vi "proba_3.vi"() -> ()   [LabVIEW 2015]
uses:
  <vilib>/MakerHub/LINX/Public/Peripherals/Digital/Digital Write N Chans.vi
  <vilib>/MakerHub/LINX/Public/Peripherals/Analog/Analog Read 1 Chan.vi
  <vilib>/MakerHub/LINX/Private/Local IO/LinxDigitalWrite.vi
  <vilib>/MakerHub/LINX/Public/Utilities/Check Channel.vi
  <vilib>/MakerHub/LINX/Public/Peripherals/Analog/Analog Read N Chans.vi
  <vilib>/MakerHub/LINX/Private/Local IO/LinxAnalogRead.vi
  <vilib>/MakerHub/LINX/Public/Utilities/Open Serial.vi
  <vilib>/MakerHub/LINX/Private/Utilties/Generate Error.vi
  <vilib>/MakerHub/LINX/LMH-LINX.lvlib
panel:
  out "x-y":u32
  out "appended array":bool[](array[boolean])
  in  "Stop Button":bool
  in  "Sample_1 (time)":dbl[][](array[numeric])
  in  "stop":bool
  in  "Sample_2 (time)":dbl[][](array[numeric])
  in  "Sample_3 (time)":dbl[][](array[numeric])
  in  "Sample_4 (time)":dbl[][](array[numeric])
  in  "LED_5 (time)":dbl[][](array[numeric])
  in  "Temp/Gap_1 (time)":dbl[][](array[numeric])
  in  "Temp/Gap_2 (time)":dbl[][](array[numeric])
  in  "Temp/Gap_3 (time)":dbl[][](array[numeric])
  in  "Temp/Gap_4 (time) 2":dbl[][](array[numeric])
  out "Ref":dbl(graph)
  in  "LED":refnum<visa-resource-name>="N/A"
  out "3":dbl(graph)
  out "2":dbl(graph)
  out "4":dbl(graph)
  out "1":dbl(graph)
  in  "milliseconds to wait":u32
  in  "Serial Port Analog":refnum<visa-resource-name>="N/A"
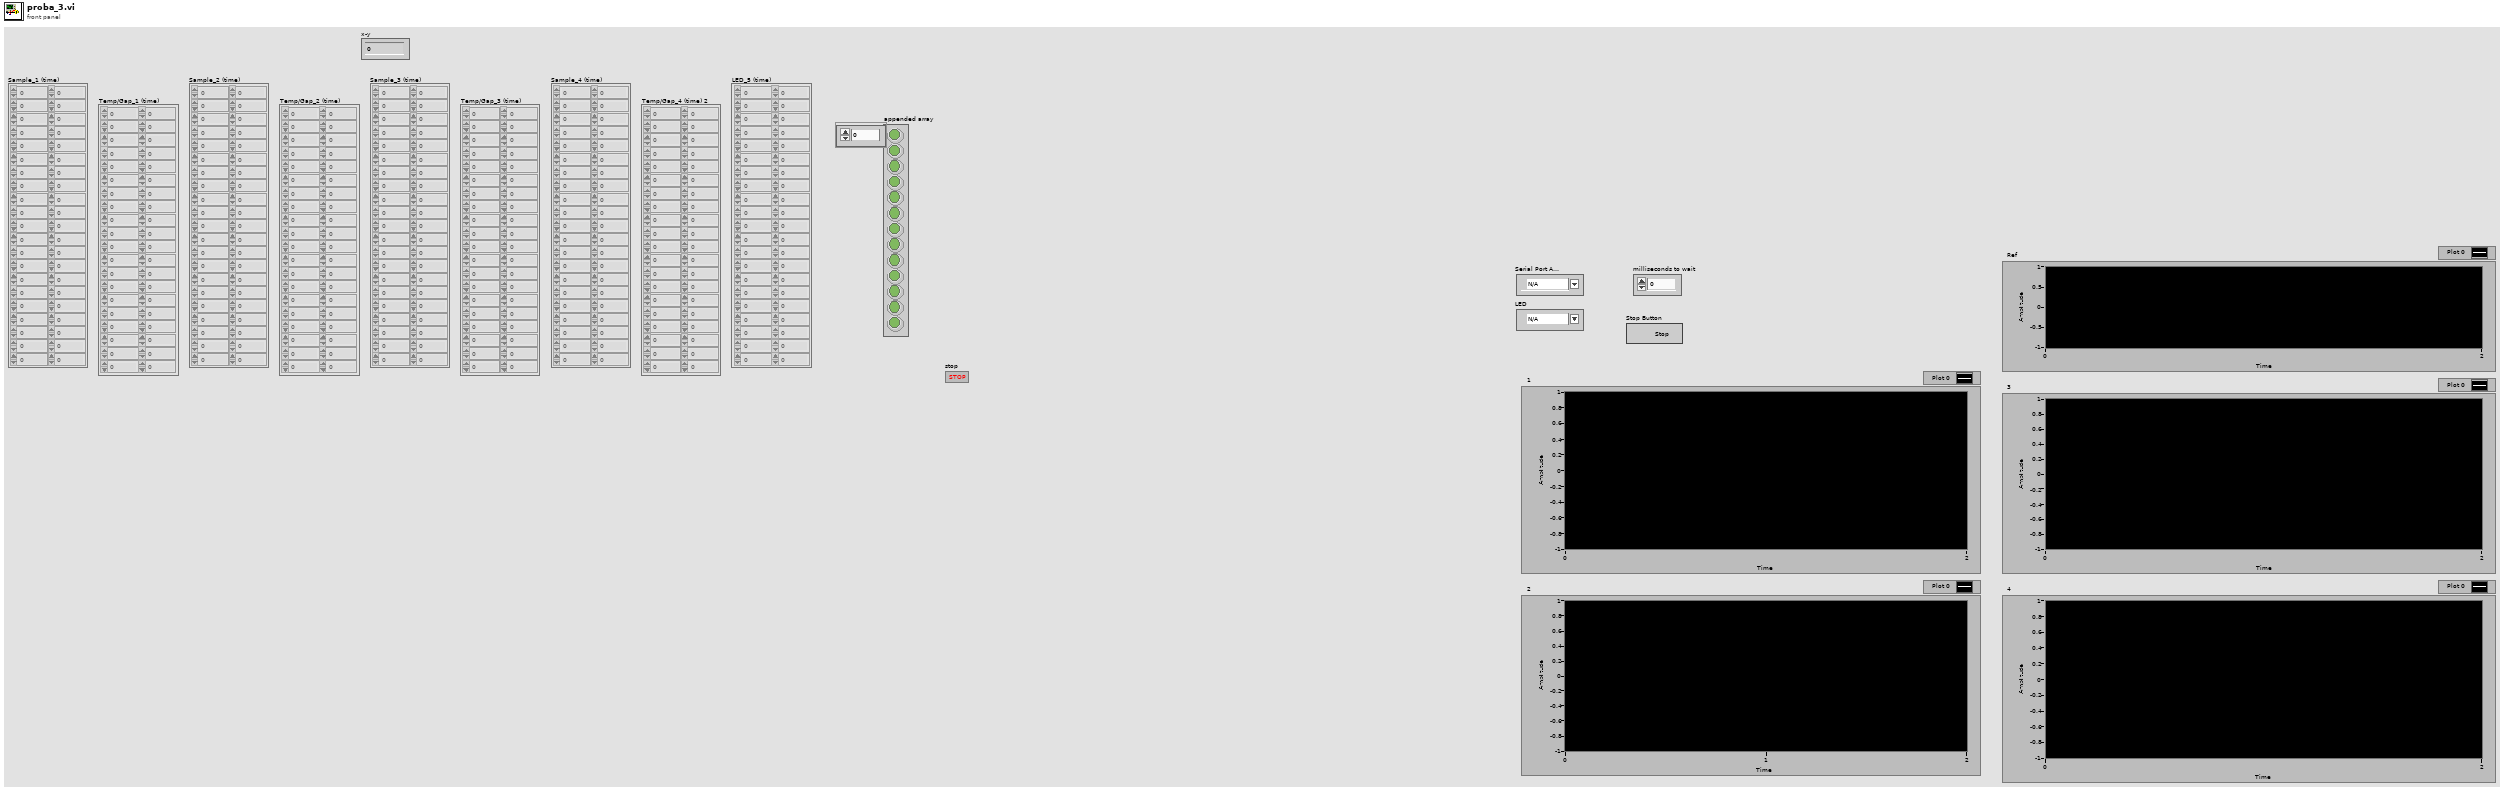
[diagram p1: front panel]
types:
  T1 = enum16{"open", "replace", "create", "open or create", "replace or create", "replace or create with confirmation"}
  T2 = typedef "LMH-LINX.lvlib/LINX Ref.ctl" = cluster{"IO":T3, "Interface":T4, "LINX Device Config":T5}
  T3 = typedef "LMH-LINX.lvlib/Platform.ctl" = enum16{"Remote", "Local"}
  T4 = typedef "LMH-LINX.lvlib/Interface.ctl" = enum16{"Serial", "TCP"}
  T5 = typedef "LMH-LINX.lvlib/Device.lvlib/LINX Device Config.ctl" = cluster{"Interface":T4, "COM Port":refnum<visa-resource-name>, "TCP Configuration":T6, "Device Family":u8, "Device ID":u8, "Device Name":string, "TCP Ref":refnum<k5>, "Channels":T7}
  T6 = typedef "LMH-LINX.lvlib/Device.lvlib/TCP Config.ctl" = cluster{"IP Address":string, "Port":u16}
  T7 = typedef "LMH-LINX.lvlib/Channels.ctl" = cluster{"DI":u8[], "DO":u8[], "AI":u8[], "AO":u8[], "PWM":u8[], "QE":u8[], "UART":u8[], "I2C 2":u8[], "SPI":u8[], "CAN":u8[], "Servo":u8[], "AI Ref (V)":dbl, "AI Resolution (Bits)":u8, "AO Ref (V)":dbl, "AO Resolution (Bits)":u8}
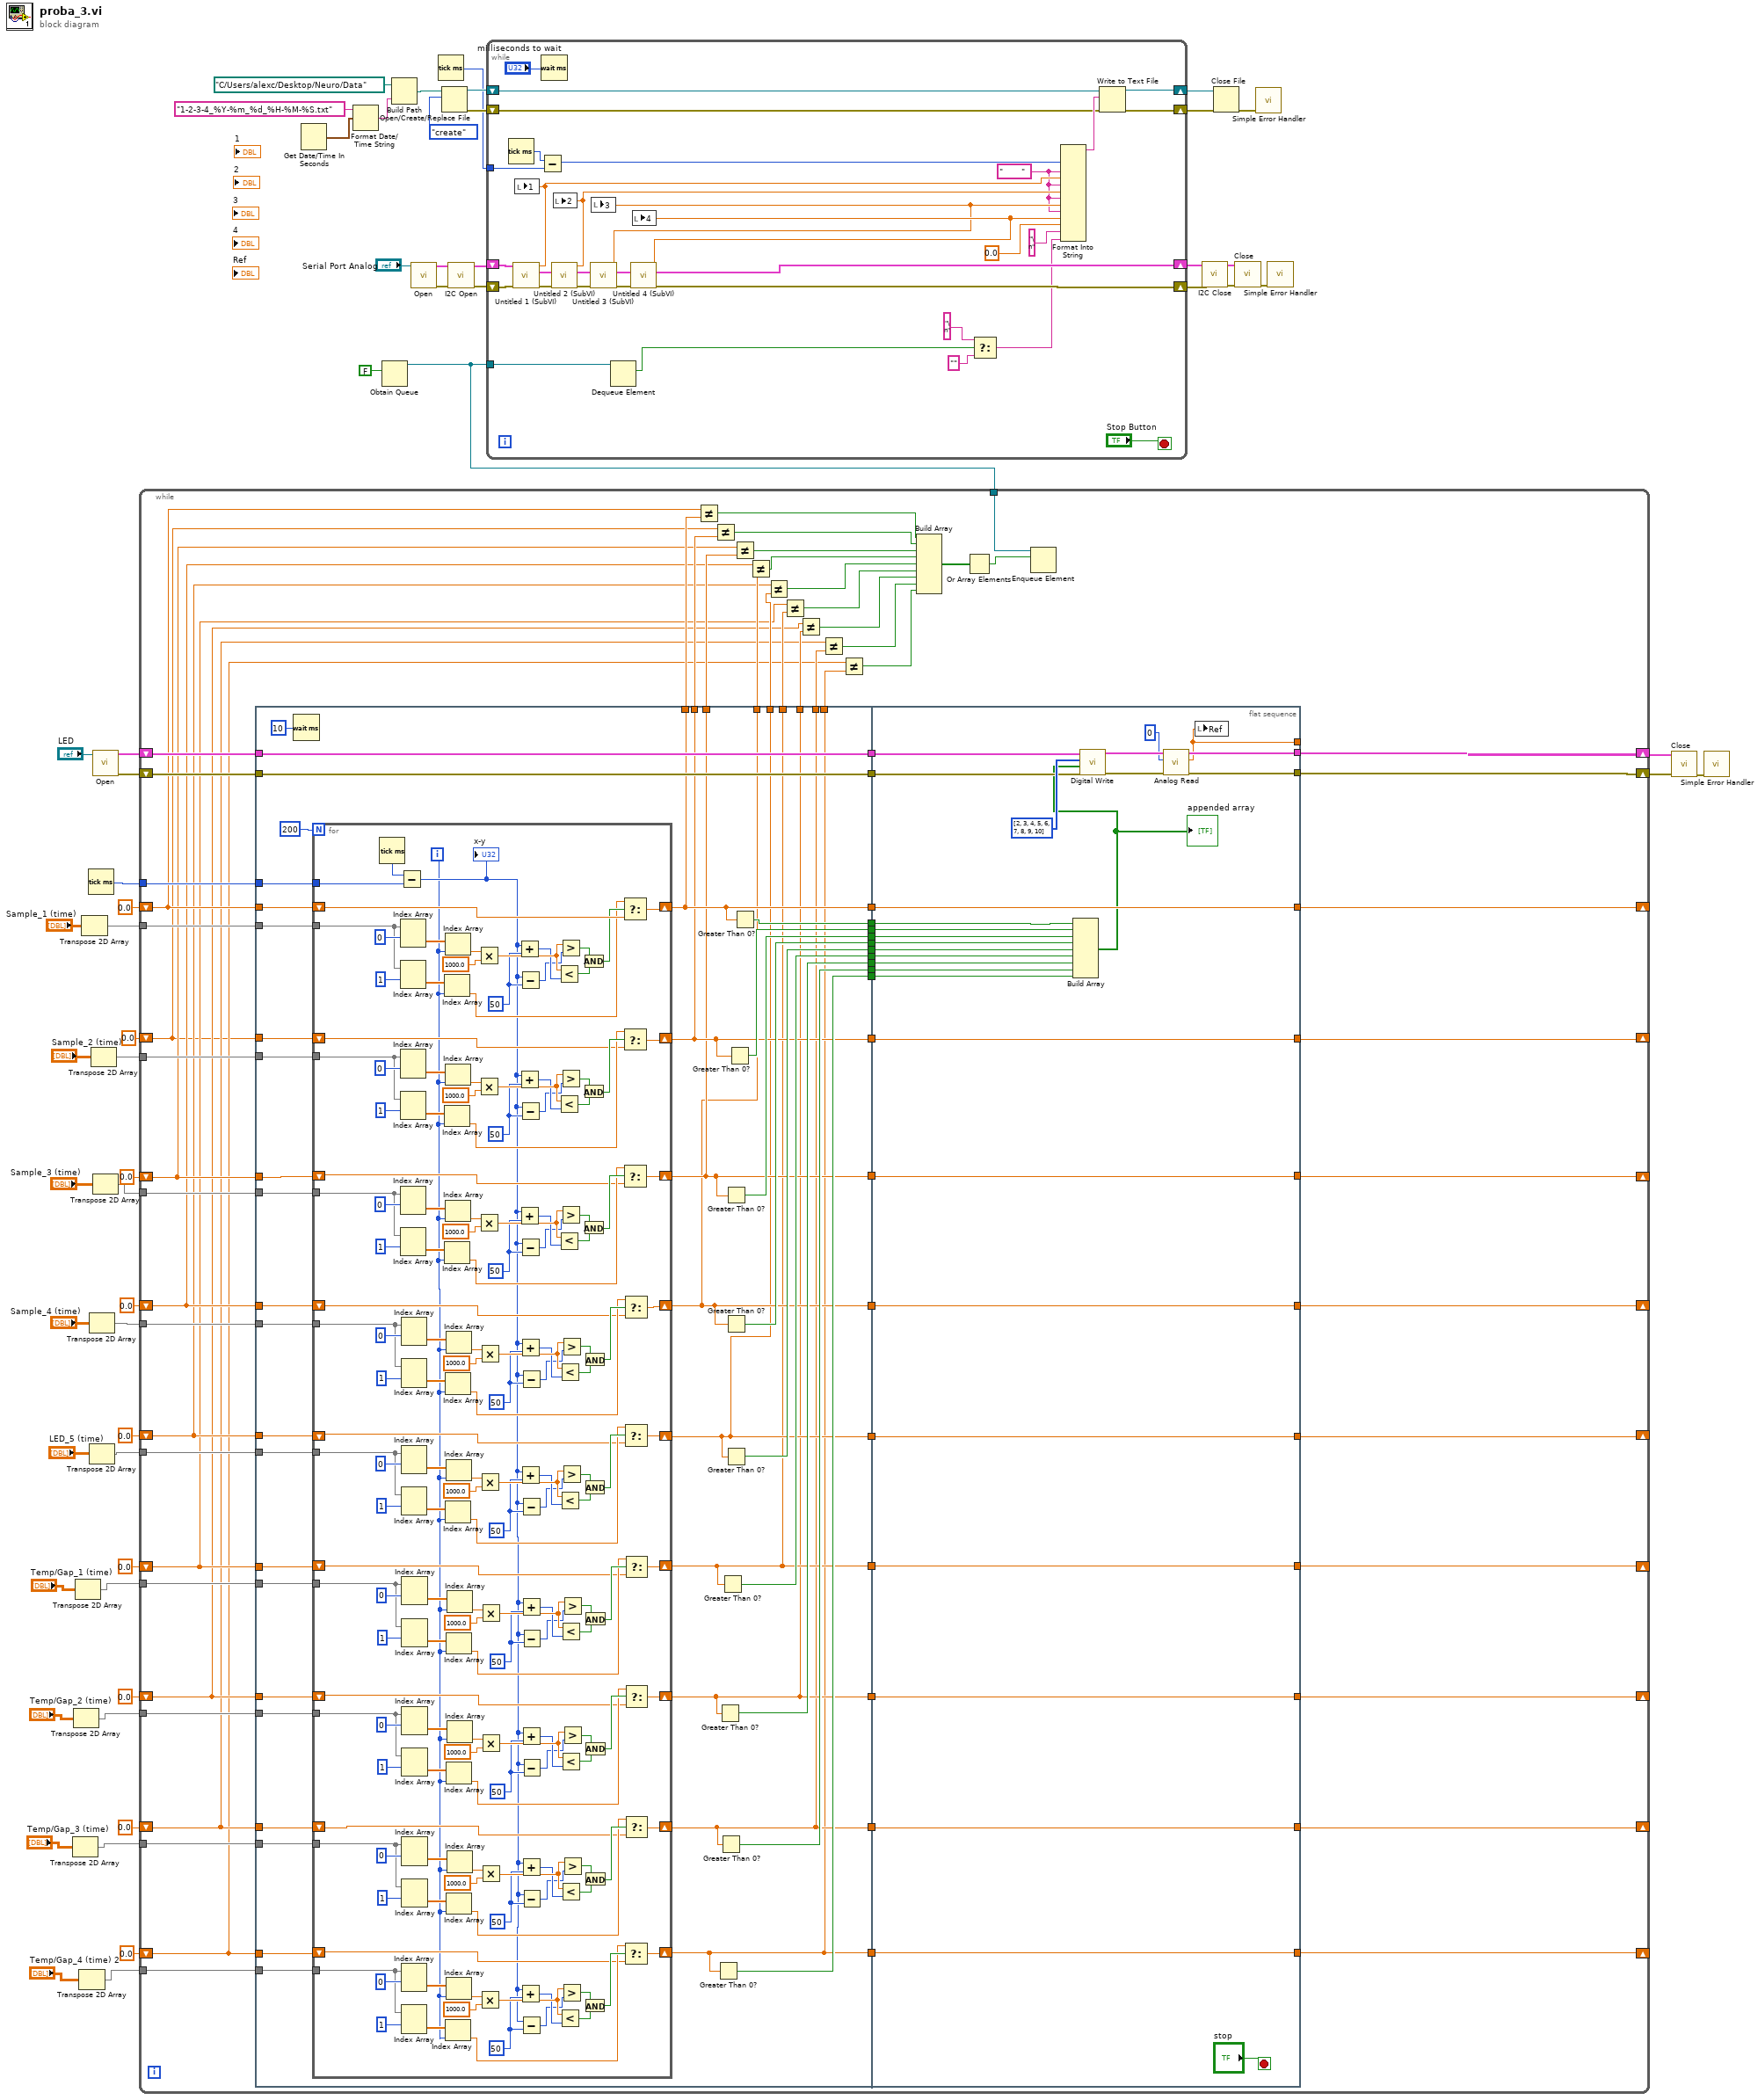
[diagram p0: block diagram]
diagram:
  n1 = Transpose 2D Array(2D array="Temp/Gap_3 (time)") -> (transposed array=w13:dbl[][])
  n2 = Transpose 2D Array(2D array="Temp/Gap_2 (time)") -> (transposed array=w14:dbl[][])
  n3 = Transpose 2D Array(2D array="Temp/Gap_1 (time)") -> (transposed array=w15:dbl[][])
  n4 = Transpose 2D Array(2D array="Temp/Gap_4 (time) 2") -> (transposed array=w12:dbl[][])
  n5 = Transpose 2D Array(2D array="Sample_1 (time)") -> (transposed array=w28:dbl[][])
  n6 = Tick Count (ms)() -> (millisecond timer value=w32:u32)
  n7 = Transpose 2D Array(2D array="Sample_4 (time)") -> (transposed array=w17:dbl[][])
  n8 = Transpose 2D Array(2D array="LED_5 (time)") -> (transposed array=w16:dbl[][])
  n9 = Transpose 2D Array(2D array="Sample_2 (time)") -> (transposed array=w26:dbl[][])
  n10 = call-poly <vilib>:"Open.vi"("Serial Port"="LED") -> ("Error Out"=w33:errorcluster, "LINX Resource"=w34:T2)  [unwired: 8 in, 1 out]
  n11 = Transpose 2D Array(2D array="Sample_3 (time)") -> (transposed array=w18:dbl[][])
  n12 = Get Date/Time In Seconds() -> (seconds since 1Jan1904=w51:timestamp)
  n13 = Format Date/Time String(time format string (%c)="1-2-3-4_%Y-%m_%d_%H-%M-%S.txt", seconds (now)=w51) -> (date/time string=w53:string)  [unwired: 1 in]
  n14 = Obtain Queue(element data type=FALSE) -> (queue out=w2:refnum<queue>)  [unwired: 4 in, 2 out]
  n15 = while {
    tunnel: w32 -> [w89]
    shift-right: [w90] -> _
    shift-left: 0.0 ("Numeric") -> [w87]
    shift-right: [w96] -> w31
    shift-left: w34 -> [w93]
    shift-right: [w95] -> w30
    shift-left: w33 -> [w91]
    tunnel: w28 -> [w131]
    tunnel: w26 -> [w130]
    shift-right: [w115] -> _
    shift-left: 0.0 ("Numeric") -> [w59]
    tunnel: w13 -> [w129]
    tunnel: w18 -> [w128]
    tunnel: w17 -> [w127]
    tunnel: w16 -> [w126]
    tunnel: w15 -> [w125]
    tunnel: w14 -> [w124]
    tunnel: w12 -> [w123]
    shift-right: [w116] -> _
    shift-left: 0.0 ("Numeric") -> [w84]
    shift-right: [w117] -> _
    shift-left: 0.0 ("Numeric") -> [w82]
    shift-right: [w118] -> _
    shift-left: 0.0 ("Numeric") -> [w80]
    shift-right: [w120] -> _
    shift-left: 0.0 ("Numeric") -> [w78]
    shift-right: [w121] -> _
    shift-left: 0.0 ("Numeric") -> [w76]
    shift-right: [w122] -> _
    shift-left: 0.0 ("Numeric") -> [w74]
    shift-right: [w119] -> _
    shift-left: 0.0 ("Numeric") -> [w72]
    tunnel: w2 -> [w60]
    stop <- "stop" stop-if-true
    n16 = flat-sequence {
      tunnel: w87 -> [w173]
      tunnel: w89 -> [w172]
      tunnel: w131 -> [w171]
      tunnel: w130 -> [w168]
      tunnel: w59 -> [w167]
      tunnel: w129 -> [w166]
      tunnel: w128 -> [w165]
      tunnel: w127 -> [w164]
      tunnel: w126 -> [w163]
      tunnel: w125 -> [w162]
      tunnel: w124 -> [w161]
      tunnel: w123 -> [w160]
      tunnel: w84 -> [w159]
      tunnel: w82 -> [w158]
      tunnel: w80 -> [w157]
      tunnel: w78 -> [w156]
      tunnel: w76 -> [w155]
      tunnel: w74 -> [w154]
      tunnel: w72 -> [w153]
      tunnel: [w134] -> w114
      tunnel: [w135] -> w113
      tunnel: [w136] -> w112
      tunnel: [w133] -> w111
      tunnel: [w137] -> w110
      tunnel: [w138] -> w109
      tunnel: [w139] -> w108
      tunnel: [w140] -> w107
      tunnel: [w141] -> w106
      tunnel: [w152] -> w105
      tunnel: [w151] -> w104
      tunnel: [w150] -> w103
      tunnel: [w149] -> w102
      tunnel: [w148] -> w101
      tunnel: [w147] -> w100
      tunnel: [w146] -> w99
      tunnel: [w145] -> w98
      tunnel: [w144] -> w97
      tunnel: [w143] -> w94
      tunnel: w93 -> [w143]
      tunnel: [w142] -> w92
      tunnel: w91 -> [w142]
      tunnel: [w141] -> w88
      tunnel: [w140] -> w86
      tunnel: [w139] -> w85
      tunnel: [w138] -> w83
      tunnel: [w137] -> w81
      tunnel: [w136] -> w79
      tunnel: [w135] -> w77
      tunnel: [w134] -> w75
      tunnel: [w133] -> w73
      tunnel: [w351] -> w115
      tunnel: [w352] -> w116
      tunnel: [w353] -> w117
      tunnel: [w354] -> w118
      tunnel: [w355] -> w119
      tunnel: [w356] -> w120
      tunnel: [w357] -> w121
      tunnel: [w358] -> w122
      tunnel: w114 -> [w358]
      tunnel: w113 -> [w357]
      tunnel: w112 -> [w356]
      tunnel: w111 -> [w355]
      tunnel: w110 -> [w354]
      tunnel: w109 -> [w353]
      tunnel: w108 -> [w352]
      tunnel: w107 -> [w351]
      tunnel: w106 -> [w346]
      tunnel: w105 -> [w342]
      tunnel: w104 -> [w341]
      tunnel: w103 -> [w340]
      tunnel: w102 -> [w339]
      tunnel: w101 -> [w338]
      tunnel: w100 -> [w337]
      tunnel: w99 -> [w336]
      tunnel: w98 -> [w335]
      tunnel: w97 -> [w345]
      tunnel: [w346] -> w90
      tunnel: [w344] -> w96
      tunnel: [w343] -> w95
      tunnel: w94 -> [w334]
      tunnel: w92 -> [w333]
      tunnel: [w331] -> _
      frame #0 {
        n17 = Wait (ms)(milliseconds to wait=u32 10) -> ()  [unwired: 1 out]
        n18 = for {
          N: 200 -> [_]
          tunnel: w172 -> [w330]
          shift-right: [w329] -> w141
          shift-left: w173 -> [w328]
          tunnel: w171 -> [w322]
          shift-right: [w297] -> w140
          shift-left: w167 -> [w296]
          tunnel: w168 -> [w295]
          shift-right: [w266] -> w139
          shift-left: w159 -> [w265]
          shift-right: [w264] -> w138
          shift-left: w158 -> [w263]
          shift-right: [w192] -> w137
          shift-left: w157 -> [w191]
          shift-right: [w189] -> w136
          shift-left: w156 -> [w190]
          shift-right: [w188] -> w135
          shift-left: w155 -> [w187]
          shift-right: [w185] -> w134
          shift-left: w154 -> [w186]
          shift-right: [w183] -> w133
          shift-left: w153 -> [w184]
          tunnel: w166 -> [w181]
          tunnel: w165 -> [w180]
          tunnel: w164 -> [w179]
          tunnel: w163 -> [w178]
          tunnel: w162 -> [w177]
          tunnel: w161 -> [w176]
          tunnel: w160 -> [w175]
          i -> [w174]
          w197 = u32 50 ("y")
          w211 = u32 50 ("y")
          w225 = u32 50 ("y")
          w239 = u32 50 ("y")
          w253 = u32 50 ("y")
          w271 = u32 50 ("y")
          w285 = u32 50 ("y")
          w302 = u32 50 ("y")
          w316 = u32 50 ("y")
          n19 = Tick Count (ms)() -> (millisecond timer value=w327:u32)
          n20 = Subtract(x=w327, y=w330) -> (x-y=w182:u32)
          "x-y" <- w182
          n21 = Index Array(array=w322, index (row)=0) -> (element=w324:dbl[])  [unwired: 1 in]
          n22 = Index Array(array=w322, index (row)=1) -> (element=w323:dbl[])  [unwired: 1 in]
          n23 = Index Array(array=w295, index (row)=0) -> (element=w309:dbl[])  [unwired: 1 in]
          n24 = Index Array(array=w295, index (row)=1) -> (element=w308:dbl[])  [unwired: 1 in]
          n25 = Index Array(array=w180, index (row)=0) -> (element=w292:dbl[])  [unwired: 1 in]
          n26 = Index Array(array=w180, index (row)=1) -> (element=w291:dbl[])  [unwired: 1 in]
          n27 = Index Array(array=w179, index (row)=0) -> (element=w278:dbl[])  [unwired: 1 in]
          n28 = Index Array(array=w179, index (row)=1) -> (element=w277:dbl[])  [unwired: 1 in]
          n29 = Index Array(array=w178, index (row)=0) -> (element=w260:dbl[])  [unwired: 1 in]
          n30 = Index Array(array=w178, index (row)=1) -> (element=w259:dbl[])  [unwired: 1 in]
          n31 = Index Array(array=w175, index (row)=0) -> (element=w204:dbl[])  [unwired: 1 in]
          n32 = Index Array(array=w175, index (row)=1) -> (element=w203:dbl[])  [unwired: 1 in]
          n33 = Index Array(array=w177, index (row)=0) -> (element=w246:dbl[])  [unwired: 1 in]
          n34 = Index Array(array=w177, index (row)=1) -> (element=w245:dbl[])  [unwired: 1 in]
          n35 = Index Array(array=w176, index (row)=0) -> (element=w232:dbl[])  [unwired: 1 in]
          n36 = Index Array(array=w176, index (row)=1) -> (element=w231:dbl[])  [unwired: 1 in]
          n37 = Index Array(array=w181, index (row)=0) -> (element=w218:dbl[])  [unwired: 1 in]
          n38 = Index Array(array=w181, index (row)=1) -> (element=w217:dbl[])  [unwired: 1 in]
          n39 = Index Array(array=w323, index=w174) -> (element=w312:dbl)
          n40 = Index Array(array=w308, index=w174) -> (element=w298:dbl)
          n41 = Index Array(array=w291, index=w174) -> (element=w281:dbl)
          n42 = Index Array(array=w324, index=w174) -> (element=w321:dbl)
          n43 = Index Array(array=w309, index=w174) -> (element=w307:dbl)
          n44 = Index Array(array=w292, index=w174) -> (element=w290:dbl)
          n45 = Index Array(array=w277, index=w174) -> (element=w267:dbl)
          n46 = Index Array(array=w259, index=w174) -> (element=w249:dbl)
          n47 = Index Array(array=w203, index=w174) -> (element=w193:dbl)
          n48 = Index Array(array=w278, index=w174) -> (element=w276:dbl)
          n49 = Index Array(array=w260, index=w174) -> (element=w258:dbl)
          n50 = Index Array(array=w245, index=w174) -> (element=w235:dbl)
          n51 = Index Array(array=w231, index=w174) -> (element=w221:dbl)
          n52 = Index Array(array=w217, index=w174) -> (element=w207:dbl)
          n53 = Index Array(array=w204, index=w174) -> (element=w202:dbl)
          n54 = Index Array(array=w246, index=w174) -> (element=w244:dbl)
          n55 = Index Array(array=w232, index=w174) -> (element=w230:dbl)
          n56 = Index Array(array=w218, index=w174) -> (element=w216:dbl)
          n57 = Multiply(x=w321, y=1000.0) -> (x*y=w317:dbl)
          n58 = Multiply(x=w307, y=1000.0) -> (x*y=w303:dbl)
          n59 = Multiply(x=w290, y=1000.0) -> (x*y=w286:dbl)
          n60 = Multiply(x=w276, y=1000.0) -> (x*y=w272:dbl)
          n61 = Multiply(x=w258, y=1000.0) -> (x*y=w254:dbl)
          n62 = Multiply(x=w202, y=1000.0) -> (x*y=w198:dbl)
          n63 = Multiply(x=w244, y=1000.0) -> (x*y=w240:dbl)
          n64 = Multiply(x=w230, y=1000.0) -> (x*y=w226:dbl)
          n65 = Multiply(x=w216, y=1000.0) -> (x*y=w212:dbl)
          n66 = Add(x=w182, y=w316) -> (x+y=w315:u32)
          n67 = Add(x=w182, y=w302) -> (x+y=w301:u32)
          n68 = Add(x=w182, y=w285) -> (x+y=w284:u32)
          n69 = Subtract(x=w182, y=w316) -> (x-y=w314:u32)
          n70 = Subtract(x=w182, y=w302) -> (x-y=w300:u32)
          n71 = Subtract(x=w182, y=w285) -> (x-y=w283:u32)
          n72 = Add(x=w182, y=w271) -> (x+y=w270:u32)
          n73 = Add(x=w182, y=w253) -> (x+y=w252:u32)
          n74 = Add(x=w182, y=w197) -> (x+y=w196:u32)
          n75 = Subtract(x=w182, y=w271) -> (x-y=w269:u32)
          n76 = Subtract(x=w182, y=w253) -> (x-y=w251:u32)
          n77 = Add(x=w182, y=w239) -> (x+y=w238:u32)
          n78 = Add(x=w182, y=w225) -> (x+y=w224:u32)
          n79 = Add(x=w182, y=w211) -> (x+y=w210:u32)
          n80 = Subtract(x=w182, y=w197) -> (x-y=w195:u32)
          n81 = Subtract(x=w182, y=w239) -> (x-y=w237:u32)
          n82 = Subtract(x=w182, y=w225) -> (x-y=w223:u32)
          n83 = Subtract(x=w182, y=w211) -> (x-y=w209:u32)
          n84 = Less?(x=w317, y=w315) -> (x < y?=w319:bool)
          n85 = Less?(x=w303, y=w301) -> (x < y?=w305:bool)
          n86 = Less?(x=w286, y=w284) -> (x < y?=w288:bool)
          n87 = Less?(x=w272, y=w270) -> (x < y?=w274:bool)
          n88 = Less?(x=w254, y=w252) -> (x < y?=w256:bool)
          n89 = Less?(x=w198, y=w196) -> (x < y?=w200:bool)
          n90 = Greater?(x=w317, y=w314) -> (0:w320:bool)
          n91 = Greater?(x=w303, y=w300) -> (0:w306:bool)
          n92 = Greater?(x=w286, y=w283) -> (0:w289:bool)
          n93 = Less?(x=w240, y=w238) -> (x < y?=w242:bool)
          n94 = Less?(x=w226, y=w224) -> (x < y?=w228:bool)
          n95 = Less?(x=w212, y=w210) -> (x < y?=w214:bool)
          n96 = Greater?(x=w272, y=w269) -> (0:w275:bool)
          n97 = Greater?(x=w254, y=w251) -> (0:w257:bool)
          n98 = Greater?(x=w198, y=w195) -> (0:w201:bool)
          n99 = Greater?(x=w240, y=w237) -> (0:w243:bool)
          n100 = Greater?(x=w226, y=w223) -> (0:w229:bool)
          n101 = Greater?(x=w212, y=w209) -> (0:w215:bool)
          n102 = And(x=w320, y=w319) -> (x .and. y?=w313:bool)
          n103 = And(x=w306, y=w305) -> (x .and. y?=w299:bool)
          n104 = And(x=w289, y=w288) -> (x .and. y?=w282:bool)
          n105 = And(x=w275, y=w274) -> (x .and. y?=w268:bool)
          n106 = And(x=w257, y=w256) -> (x .and. y?=w250:bool)
          n107 = And(x=w201, y=w200) -> (x .and. y?=w194:bool)
          n108 = And(x=w243, y=w242) -> (x .and. y?=w236:bool)
          n109 = And(x=w229, y=w228) -> (x .and. y?=w222:bool)
          n110 = And(x=w215, y=w214) -> (x .and. y?=w208:bool)
          n111 = Select(t=w312, s=w313, f=w328) -> (s? t:f=w329:dbl)
          n112 = Select(t=w298, s=w299, f=w296) -> (s? t:f=w297:dbl)
          n113 = Select(t=w281, s=w282, f=w265) -> (s? t:f=w266:dbl)
          n114 = Select(t=w267, s=w268, f=w263) -> (s? t:f=w264:dbl)
          n115 = Select(t=w249, s=w250, f=w191) -> (s? t:f=w192:dbl)
          n116 = Select(t=w193, s=w194, f=w184) -> (s? t:f=w183:dbl)
          n117 = Select(t=w235, s=w236, f=w190) -> (s? t:f=w189:dbl)
          n118 = Select(t=w221, s=w222, f=w187) -> (s? t:f=w188:dbl)
          n119 = Select(t=w207, s=w208, f=w186) -> (s? t:f=w185:dbl)
        }
        n120 = Greater Than 0?(x=w133) -> (x > 0?=w145:bool)
        n121 = Greater Than 0?(x=w135) -> (x > 0?=w147:bool)
        n122 = Greater Than 0?(x=w134) -> (x > 0?=w146:bool)
        n123 = Greater Than 0?(x=w136) -> (x > 0?=w148:bool)
        n124 = Greater Than 0?(x=w139) -> (x > 0?=w151:bool)
        n125 = Greater Than 0?(x=w138) -> (x > 0?=w150:bool)
        n126 = Greater Than 0?(x=w137) -> (x > 0?=w149:bool)
        n127 = Greater Than 0?(x=w140) -> (x > 0?=w152:bool)
        n128 = Greater Than 0?(x=w141) -> (x > 0?=w144:bool)
      }
      frame #1 {
        n129 = Build Array(w345, w342, w341, w340, w339, w338, w337, w336, w335) -> (w332:bool[])
        "appended array" <- w332
        n130 = call-poly <vilib>:"Digital Write.vi"("Error In"=w333, "Values"=w332, "DO Channels"=u8[] [2, 3, 4, 5, 6, 7, 8, 9, 10], "LINX Resource"=w334) -> ("Error Out"=w350:errorcluster, "LINX Resource"=w349:T2)  [unwired: 6 in]
        n131 = call-poly <vilib>:"Analog Read.vi"("Error In"=w350, "Analog Channel"=u8 0, "LINX Resource"=w349) -> ("Error Out"=w343:errorcluster, "Voltage"=w331:dbl, "LINX Resource"=w344:T2)  [unwired: 5 in, 1 out]
        n132 = local write "Ref"(w331) -> ()
      }
    }
    n133 = Not Equal?(x=w87, y=w88) -> (x != y?=w71:bool)
    n134 = Not Equal?(x=w59, y=w86) -> (x != y?=w70:bool)
    n135 = Not Equal?(x=w84, y=w85) -> (x != y?=w68:bool)
    n136 = Not Equal?(x=w82, y=w83) -> (x != y?=w67:bool)
    n137 = Not Equal?(x=w80, y=w81) -> (x != y?=w66:bool)
    n138 = Not Equal?(x=w78, y=w79) -> (x != y?=w65:bool)
    n139 = Not Equal?(x=w76, y=w77) -> (x != y?=w64:bool)
    n140 = Not Equal?(x=w74, y=w75) -> (x != y?=w63:bool)
    n141 = Not Equal?(x=w72, y=w73) -> (x != y?=w62:bool)
    n142 = Build Array(w71, w70, w68, w67, w66, w65, w64, w63, w62) -> (w69:bool[])
    n143 = Or Array Elements(Boolean array=w69) -> (logical OR=w61:bool)
    n144 = Enqueue Element(queue=w60, element=w61) -> ()  [unwired: 2 in, 3 out]
  }
  n145 = Build Path(base path=path "C:/Users/alexc/Desktop/Neuro/Data", name or relative path=w53) -> (appended path=w50:path)
  n146 = call-poly <vilib>:"Open.vi"("Serial Port"="Serial Port Analog") -> ("Error Out"=w57:errorcluster, "LINX Resource"=w58:T2)  [unwired: 8 in, 1 out]
  n147 = Tick Count (ms)() -> (millisecond timer value=w46:u32)
  n148 = Open/Create/Replace File(file path (use dialog)=w50, operation (0:open)=T1."create") -> (refnum out=w48:refnum<file>, error out=w47:errorcluster)  [unwired: 4 in, 1 out]
  n149 = call <vilib>:"I2C Open.vi"("Error In"=w57, "LINX Resource"=w58) -> ("Error Out"=w44:errorcluster, "LINX Resource"=w45:T2)  [unwired: 8 in]
  n150 = while {
    tunnel: w46 -> [w383]
    shift-right: [w379] -> w36
    shift-left: w48 -> [w381]
    shift-right: [w378] -> w35
    shift-left: w47 -> [w380]
    shift-right: [w375] -> w38
    shift-left: w45 -> [w377]
    shift-right: [w374] -> w37
    shift-left: w44 -> [w376]
    tunnel: w2 -> [w363]
    stop <- "Stop Button" stop-if-true
    w368 = "       "
    n151 = Tick Count (ms)() -> (millisecond timer value=w384:u32)
    n152 = call "Untitled 1 (SubVI).vi"("error in (no error)"=w376, "LINX Resource in"=w377) -> ("error out"=w389:errorcluster, "LINX Resource out"=w390:T2, "Numeric"=w372:dbl)  [unwired: 7 in]
    n153 = local write "1"(w372) -> ()
    n154 = Subtract(x=w384, y=w383) -> (x-y=w369:u32)
    n155 = Wait (ms)(milliseconds to wait="milliseconds to wait") -> ()  [unwired: 1 out]
    n156 = call "Untitled 2 (SubVI).vi"("error in (no error)"=w389, "LINX Resource in"=w390) -> ("error out"=w388:errorcluster, "LINX Resource"=w387:T2, "Numeric"=w371:dbl)  [unwired: 7 in]
    n157 = local write "2"(w371) -> ()
    n158 = call "Untitled 3 (SubVI).vi"("error in (no error)"=w388, "LINX Resource in"=w387) -> ("error out"=w385:errorcluster, "LINX Resource out"=w386:T2, "Numeric"=w370:dbl)  [unwired: 7 in]
    n159 = local write "3"(w370) -> ()
    n160 = Dequeue Element(queue=w363) -> (element=w362:bool)  [unwired: 2 in, 3 out]
    n161 = call "Untitled 4 (SubVI).vi"("error in (no error)"=w385, "LINX Resource in"=w386) -> ("error out"=w374:errorcluster, "LINX Resource"=w375:T2, "Numeric"=w373:dbl)  [unwired: 7 in]
    n162 = local write "4"(w373) -> ()
    n163 = Select(t="\n" ("input 10"), s=w362, f="") -> (s? t:f=w361:string)
    n164 = Format Into String(w369, w368, w372, w368, w371, w368, w370, w368, w373, 0.0 ("element"), "\n" ("input 10"), w361) -> (resulting string=w382:string)  [unwired: 3 in, 1 out]
    n165 = Write to Text File(file (use dialog)=w381, text=w382, error in=w380) -> (refnum out=w379:refnum<file>, error out=w378:errorcluster)  [unwired: 1 in, 1 out]
  }
  n166 = call <vilib>:"I2C Close.vi"("Error In"=w37, "LINX Resource"=w38) -> ("Error Out"=w40:errorcluster, "LINX Resource"=w41:T2)  [unwired: 8 in]
  n167 = Close File(refnum=w36, error in=w35) -> (error out=w43:errorcluster)  [unwired: 1 out]
  n168 = call <vilib>:"Close.vi"("Error In"=w40, "LINX Resource"=w41) -> ("Error Out"=w42:errorcluster)  [unwired: 9 in]
  n169 = call <vilib>:"Simple Error Handler.vi"("error in (no error)"=w43) -> ()  [unwired: 4 in, 5 out]
  n170 = call <vilib>:"Simple Error Handler.vi"("error in (no error)"=w42) -> ()  [unwired: 4 in, 5 out]
  n171 = call <vilib>:"Close.vi"("Error In"=w30, "LINX Resource"=w31) -> ("Error Out"=w39:errorcluster)  [unwired: 9 in]
  n172 = call <vilib>:"Simple Error Handler.vi"("error in (no error)"=w39) -> ()  [unwired: 4 in, 5 out]
